vi "String to Complex Number (CDB).vi"(2 "use system decimal point (T)":bool=TRUE, 3 "default (0 CDB)":cdb, 4 "offset":i32, 5 "string":string) -> (0 "number":cdb, 1 "offset past number":i32)   [LabVIEW 2018, in "Numeric Data Type.lvclass"]
doc: "<b> </b> <b> </b>\n©2013, Q Software Innovations, LLC.\n\nWritten in National Instruments LabVIEW™ 2013.\n\nAuthored by Quentin Alldredge\nQ@qsoftwareinnovations.com\nwww.qsoftwareinnovations.com\n\nAll rights reserved."
uses:
  Numeric Data Type.lvclass
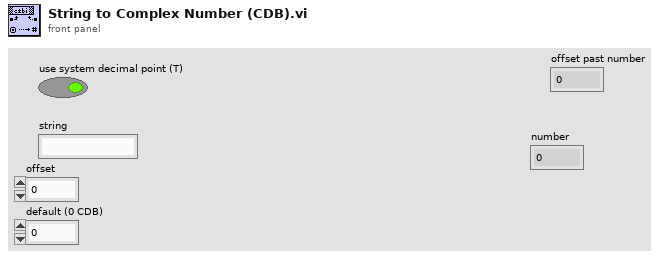
[diagram p1: front panel]
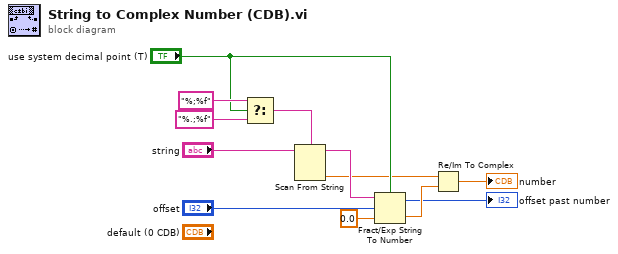
[diagram p0: block diagram]
diagram:
  n1 = Select(t="%;%f", s="use system decimal point (T)", f="%.;%f") -> (s? t:f=w10:string)
  n2 = Scan From String(format string=w10, input string="string") -> (remaining string=w8:string, output 1=w6:dbl)  [unwired: 3 in, 2 out]
  n3 = Fract/Exp String To Number(use system decimal point (T)="use system decimal point (T)", string=w8, offset="offset", default (0 dbl)=0.0 ("default (0 DBL)")) -> (offset past number=→"offset past number":i32, number=w5:dbl)
  n4 = Re/Im To Complex(1:w5, 2:w6) -> (0:→"number":cdb)
